vi "Write Msg Input.vi"(10 "Msg Input":refnum<class "Msg Input.lvclass">, 11 "Stopped Msg in":refnum<class "Stopped Msg.lvclass">) -> (3 "Stopped Msg out":refnum<class "Stopped Msg.lvclass">)   [LabVIEW 2025, in "jettl.lvlib" / "Stopped jettl Msg.lvlib" / "Stopped Msg.lvclass"]
uses:
  Stopped Msg.lvclass
  Msg Input/Msg Input.lvclass
  Stopped Msg.lvclass/Stopped Msg.ctl
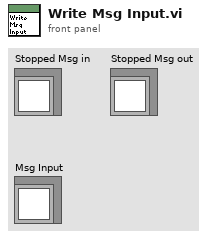
[diagram p1: front panel]
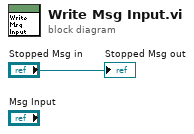
[diagram p0: block diagram]
diagram:
  "Stopped Msg out" <- "Stopped Msg in"
